vi "Error Converter.vi"(0 "error in (no error)":errorcluster, 1 "String to add to error message":string) -> (2 "error out (no error)":errorcluster)   [LabVIEW 2011]
doc: "This vi adds an arbitrary string to an error. If no error exists, the string will not be added."
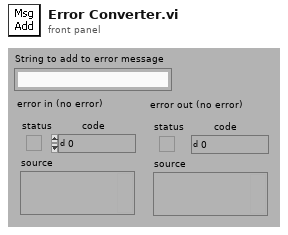
[diagram p1: front panel]
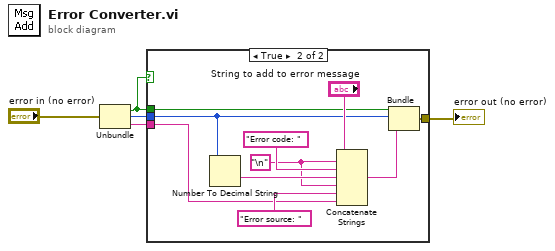
[diagram p0: block diagram]
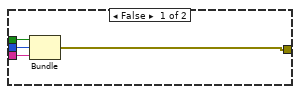
[diagram p2: hidden frame]
diagram:
  n1 = Unbundle("error in (no error)") -> ("status"=w1:bool, "code"=w4:i32, "source"=w3:string)
  n2 = case shown="True" w1 {
    tunnel: [w6 w14] -> w5
    tunnel: w1 -> [w9 w13]
    tunnel: w4 -> [w8 w12]
    tunnel: w3 -> [w7 w11]
    frame False {
      n3 = Bundle("status"=w9, "code"=w8, "source"=w7) -> (w6:errorcluster)  [unwired: 1 in]
    }
    frame True {
      w10 = "\n"
      n4 = Number To Decimal String(number=w12) -> (decimal integer string=w16:string)  [unwired: 1 in]
      n5 = Concatenate Strings("String to add to error message", w10, "Error code: " ("string"), w16, w10, "Error source: " ("string"), w11) -> (w18:string)
      n6 = Bundle("status"=w13, "code"=w12, w18) -> (w14:cluster{"status":bool, "code":i32, string})  [unwired: 1 in]
    }
  }
  "error out (no error)" <- w5
